vi "add_quote_for_str.vi"(11 "input":string) -> (3 "output":string)   [LabVIEW 2020]
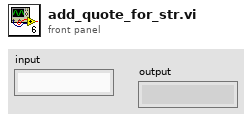
[diagram p1: front panel]
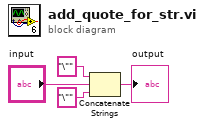
[diagram p0: block diagram]
diagram:
  n1 = Concatenate Strings("\"" ("字符串"), "input", "\"" ("字符串")) -> (→"output":string)
